vi "LabVLC - MuteControl.vi"(3 "error in (no error)":errorcluster, 4 "is_mute":bool, 5 "struct":T1={"media_ptr"=0, "vlc_inst_ptr"=0, "path in"=path "C:/Program Files (x86)/VideoLAN/VLC/libvlc.dll"}) -> (0 "error out":errorcluster, 1 "is_mute":bool, 2 "out":T1)   [LabVIEW 2014]
doc: "Mute the VLC player. If true, the video is muted. If false, the audio is playing. Use with a switch for best effect. Requires a media pointer. The ramifications of calling this function before play are unknown. You may optionally use the boolean output of the mute function to programmatically determine the state of mutes. Mute function will override volume control."
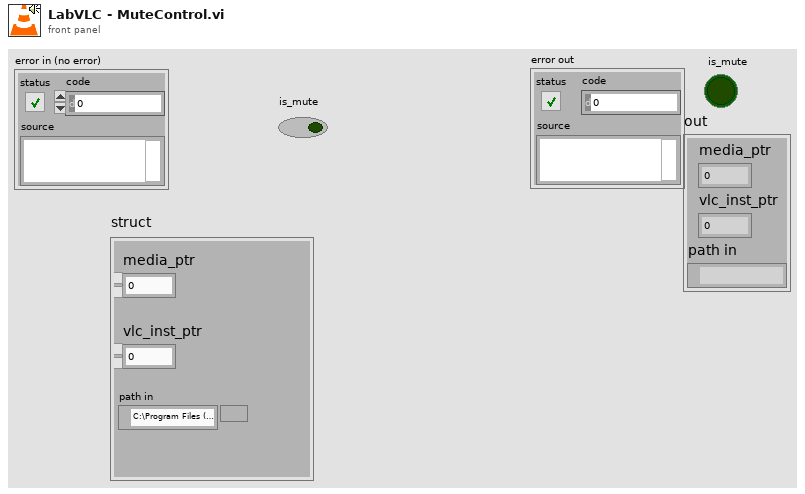
[diagram p1: front panel]
types:
  T1 = cluster{"media_ptr":i32, "vlc_inst_ptr":i32, "path in":path}
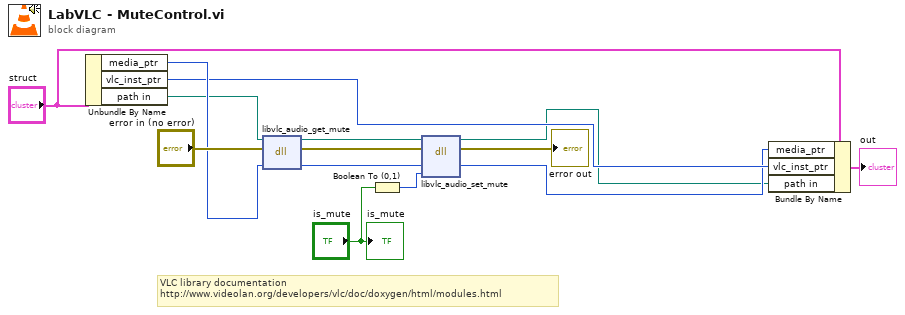
[diagram p0: block diagram]
diagram:
  # "VLC library documentation\nhttp://www.videolan.org/developers/vlc/doc/doxygen/html/modules.html"
  n1 = Unbundle By Name("struct") -> ("media_ptr"=w7:i32, "vlc_inst_ptr"=w4:i32, "path in"=w6:path)
  n2 = dll-call lib="C:/Program Files (x86)/VideoLAN/VLC/libvlc.dll" fn="libvlc_audio_get_mute"(path in=w6, error in="error in (no error)", "media_pointer"=w7) -> (path out=w8:path, error out=w12:errorcluster, "media_pointer"=w13:i32)  [unwired: 2 in]
  n3 = Boolean To (0,1)(Boolean="is_mute") -> (0, 1=w9:i16)
  n4 = dll-call lib="C:/Program Files (x86)/VideoLAN/VLC/libvlc.dll" fn="libvlc_audio_set_mute"(path in=w8, error in=w12, "media_pointer"=w13, "status"=w9) -> (path out=w2:path, error out=→"error out":errorcluster, "media_pointer"=w3:i32)  [unwired: 3 in]
  n5 = Bundle By Name(cluster="struct", "media_ptr"=w3, "vlc_inst_ptr"=w4, "path in"=w2) -> (→"out":T1)
  "is_mute" <- "is_mute"
